vi "enable_run_button.vi"(0 "Boolean":bool, 1 "Run":refnum<vi>) -> ()   [LabVIEW 2015]
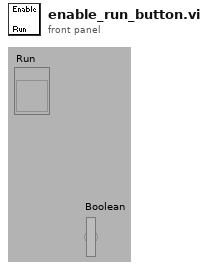
[diagram p1: front panel]
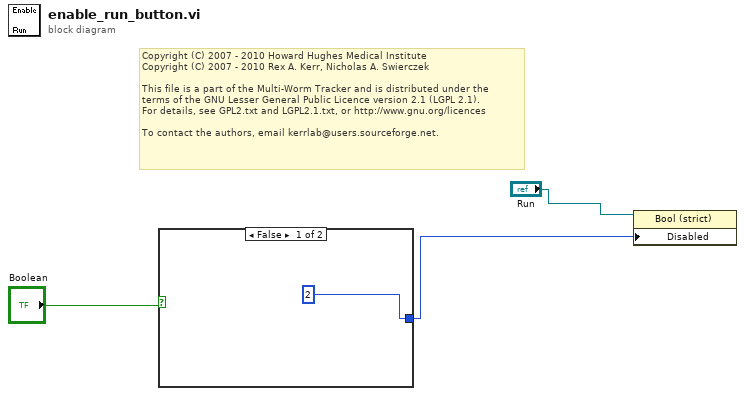
[diagram p0: block diagram]
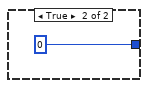
[diagram p2: hidden frame]
diagram:
  # "Copyright (C) 2007 - 2010 Howard Hughes Medical Institute\nCopyright (C) 2007 - 2010 Rex A. Kerr, Nicholas A. Swierczek\n \nThis file is a part of the Multi-Worm Tracker and is distributed under the\nterms of the GNU Lesser General Public Licence version 2.1 (LGPL 2.1).\nFor details, see GPL2.txt and LGPL2.1.txt, or http://www.gnu.org/licences\n \nTo contact the authors, email kerrlab@users.sourceforge.net."
  n1 = case shown="False" "Boolean" {
    tunnel: [2 0] -> w2
    frame False {
    }
    frame True {
    }
  }
  n2 = property class="Bool (strict)"(reference="Run", "Disabled"=w2) -> ()  [unwired: 1 in, 2 out]
